vi "LDA_Beam_Alignment.vi"() -> ()   [LabVIEW 2014]
uses:
  Anemometry Sub Vis/Controls/Beam_Type.ctl
  Anemometry Sub Vis/Gen Trav/Traverse_cluster.ctl
  Anemometry Sub Vis/Gen Trav/Spacing.ctl
  Anemometry Sub Vis/Controls/Multi_run_mode.ctl
  Anemometry Sub Vis/Controls/User_Specific_mode.ctl
  Anemometry Sub Vis/Controls/Tunnel_Coordinates.ctl
  Anemometry Sub Vis/Controls/Post_Process.ctl
  Anemometry Sub Vis/Controls/Setup.ctl
  Anemometry Sub Vis/Gen Trav/Trav_mode.ctl
  Anemometry Sub Vis/Globals/Trav_pos_global.vi
  Anemometry Sub Vis/Globals/Meas_global.vi
  Anemometry Sub Vis/Globals/Preference_global.vi
panel:
  in  "Beams to peak":bool[](array[boolean])=[TRUE, TRUE, TRUE, TRUE]
  out "Beam Names":string[](array[string])
  out "Probe is facing...":string
  out "In-Plane Roll (deg)":dbl
  out "Pitch (deg)":dbl
  out "Yaw (deg)":dbl
  out "Vp (Actual Probe dir. vect)":dbl[](array[numeric])
  in  "Mode":T1(ring)
  out "Values Out":dbl[][](array[numeric])
  out "Original Position":dbl[](array[numeric]) format="%.2f"
  in  "Traverse Position":dbl[](array[numeric])=[0.0, 0.0, 0.0] format="%.2f"
  out "Message":string
  in  "Go Back":bool
  in  "OK":bool
  in  "stop":bool
  in  "Working On":T2 items=["Green Unshifted", "Green Shifted", "Blue Unshifted", "Blue Shifted"]
  # "X                 Y              Z"
  # "X                 Y              Z"
  # "Green Unshifted\nGreen Shifted\nBlue Unshifted\nBlue Shifted"
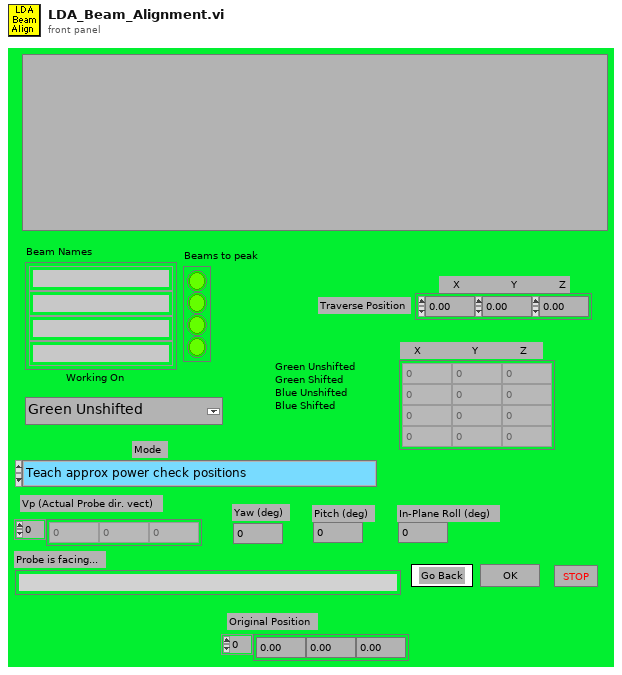
[diagram p1: front panel]
types:
  T1 = enum16{"Teach approx power check positions", "Hunt for optimum power check positions", "Check Beam powers now", "Peak up beam power using manipulators"}
  T2 = typedef "Beam_Type.ctl" = u16
  T3 = typedef "Traverse_cluster.ctl" = cluster{"Start X":dbl, "Start Y":dbl, "Start Z":dbl, "End X":dbl, "End Y":dbl, "End Z":dbl, "No. of pts.":i32, "Spacing":T4, "Filename":path, "Tunnel Speed":dbl, "Averaging time (min)":dbl, "Extra Commands":string, "Specific Arguments":string, "Emission Rate (l/min)":dbl, "Trace Gas Concentration (%)":dbl, "Density Ratio":string, "Comments":string, "Row No":i32, "Row Type Selector":T5, "Completion time":string, "Row Duration (mins)":dbl, "No. of Valid pts.":i32, "Meas Setup File":string}
  T4 = typedef "Spacing.ctl" = enum16{"Linear", "Log", "Gauss", "Specified", "N/A"}
  T5 = typedef "Multi_run_mode.ctl" = enum16{"Move Traverse Only", "Set Tunnel Speed Only", "Set Source Only", "Set Measurement Conditions", "Single Measurement", "Vertical Profile", "Lateral Profile", "Longitudinal Profile", "Explore Volume", "Multi-Axis Profile", "Auto Calibrate", "Meas Fast FID Bkgnd", "Check Beam Power", "Scanning Valve Measurement", "Run VI Named:", "Set ADAM Ch", "Wait (minutes)", "Send Message", "Synchronize With:", "Fall Back to this Row", "Turn Off Row Repeating", "Blank Row", "Traverse 3D Volume"}
  T6 = typedef "Tunnel_Coordinates.ctl" = enum16{"Work in Tunnel Coordinates", "Work in Model Coordinates"}
  T7 = typedef "User_Specific_mode.ctl" = enum16{"Check VI only", "Run VI"}
  T8 = typedef "Post_Process.ctl" = enum16{"Take New Data", "Post Process Raw Data File"}
  T9 = enum16{"Load setup from excel file", "Save setup to excel file"}
  T10 = enum16{"Load From Excel File", "Save to Excel File"}
  T11 = typedef "Setup.ctl" = enum16{"Run Program", "Show Setup", "Save Current Setup", "Setup Front Panel"}
  T12 = typedef "Trav_mode.ctl" = enum16{"Move traverse", "Read traverse position", "Teach Position"}
  T13 = typedef "LDA_Beam_Cluster.ctl" = cluster{"Vg1 (Green 1 dir. vect.)":dbl[], "Vg2  (Green 2 dir. vect.)":dbl[], "Vb1 (Blue 1 dir. vect.)":dbl[], "Vb2 (Blue 1 dir. vect.)":dbl[], "Porb (Orb XYZ posn. forced coplanar)":dbl[], "Porb (Orb XYZ posn. - allow skew)":dbl[], "Orb posn. uncertainty, +/- dx, dy, dz":dbl[], "Vp (Actual Probe dir. vect)":dbl[], "Yaw (deg)":dbl, "Pitch (deg)":dbl, "In-Plane Roll (deg)":dbl, "Beam Half Angle (deg)":dbl, "B1 Close P11":dbl[], "B1 Far P12":dbl[], "B2 Close P22":dbl[], "B2 Far P21":dbl[], "Projected Roll (deg)":dbl, "Green Velocity Vector":dbl[], "Blue Velocity Vector":dbl[], "Probe is facing....":string, "Calculation Method":string}
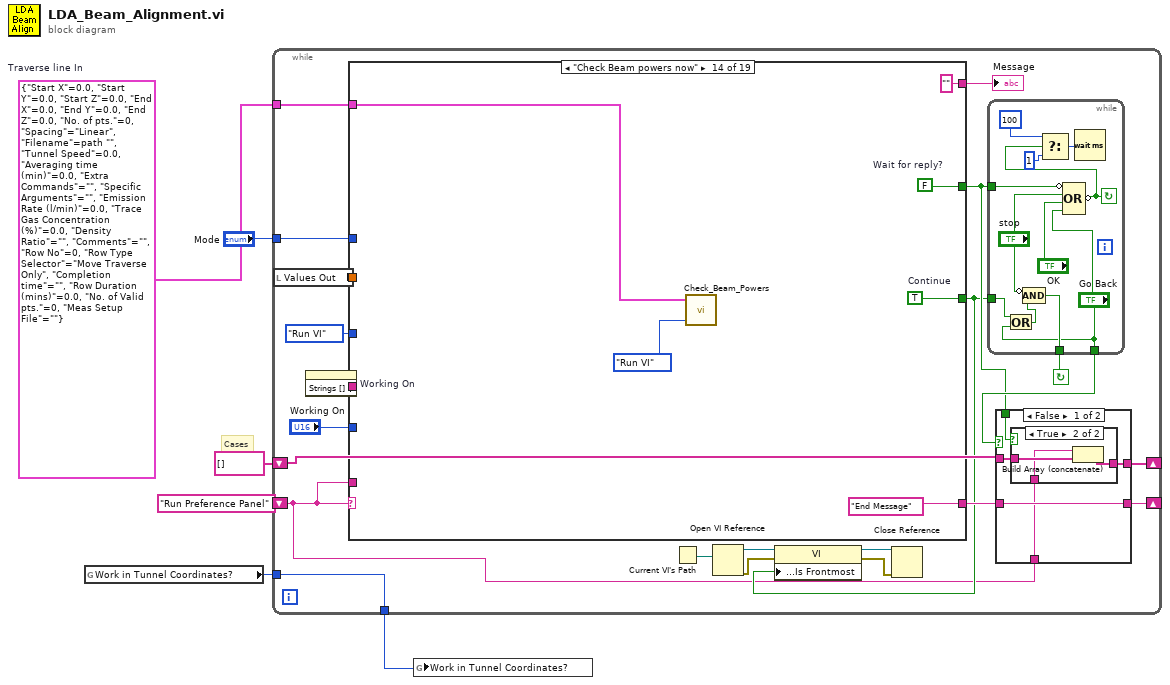
[diagram p0: block diagram]
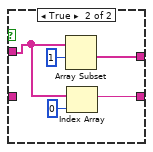
[diagram p3: hidden frame]
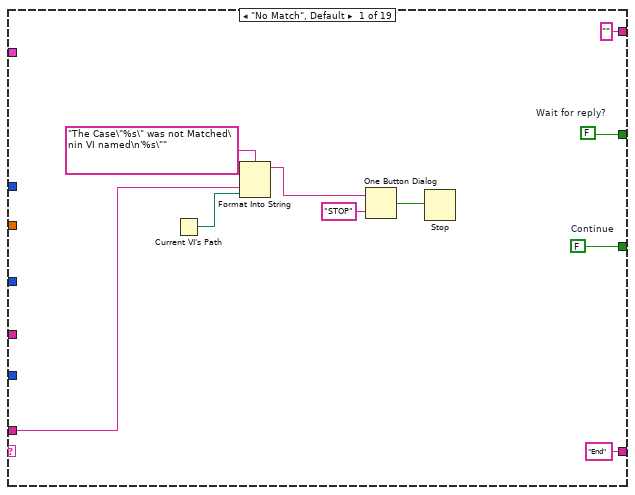
[diagram p4: hidden frame]
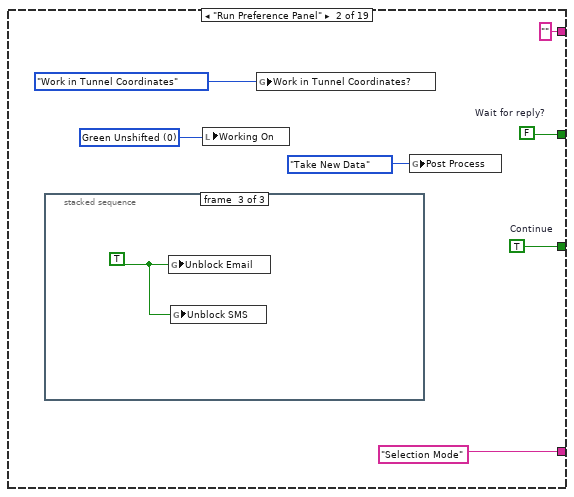
[diagram p5: hidden frame]
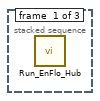
[diagram p6: hidden frame]
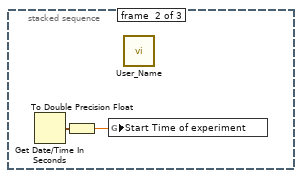
[diagram p7: hidden frame]
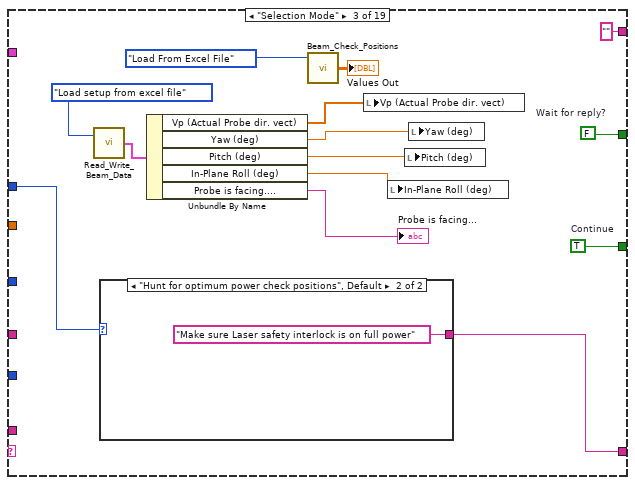
[diagram p8: hidden frame]
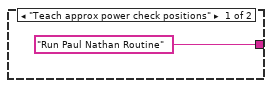
[diagram p9: hidden frame]
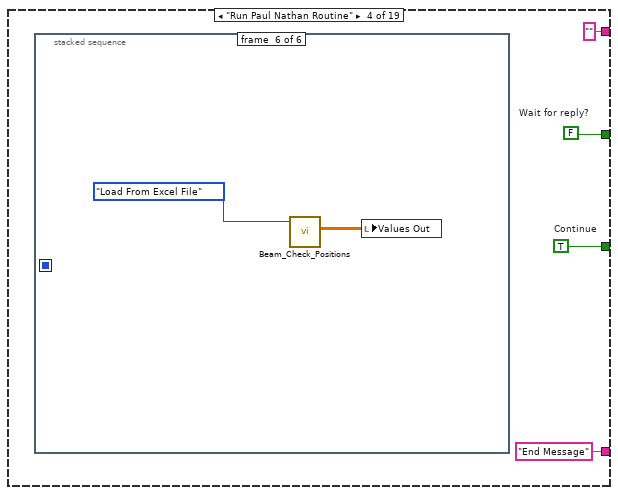
[diagram p10: hidden frame]
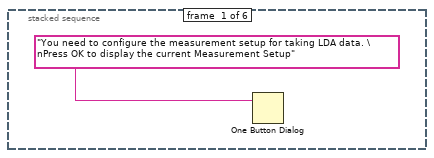
[diagram p11: hidden frame]
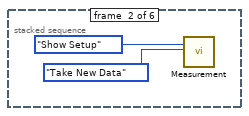
[diagram p12: hidden frame]
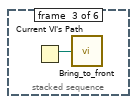
[diagram p13: hidden frame]
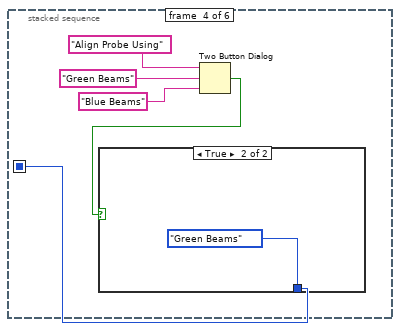
[diagram p14: hidden frame]
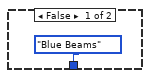
[diagram p15: hidden frame]
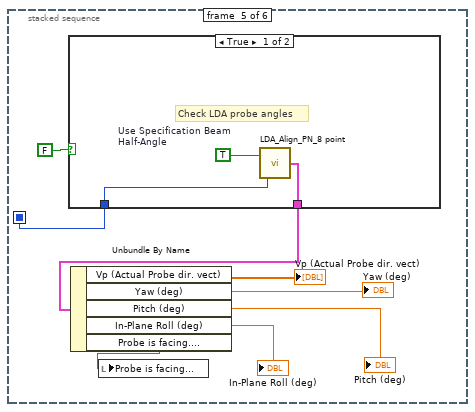
[diagram p16: hidden frame]
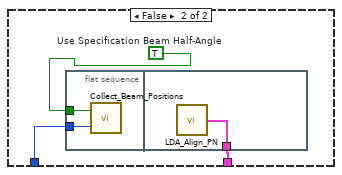
[diagram p17: hidden frame]
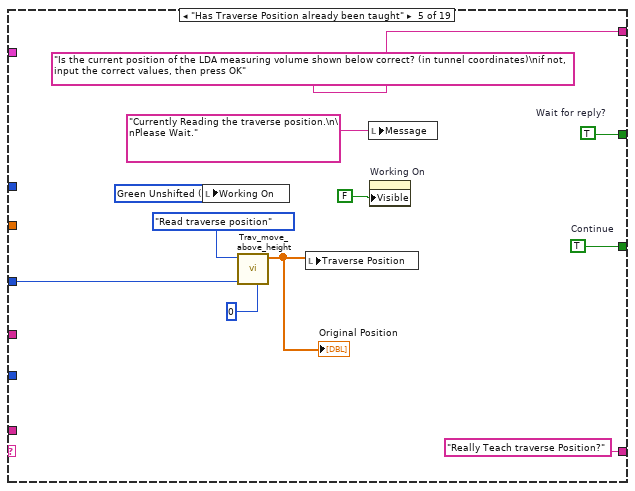
[diagram p18: hidden frame]
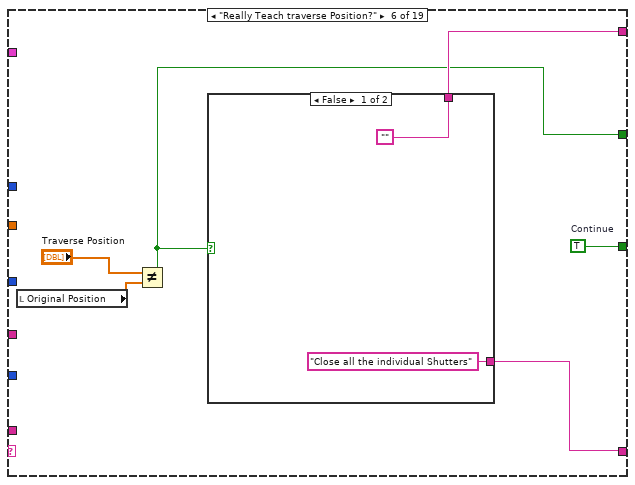
[diagram p19: hidden frame]
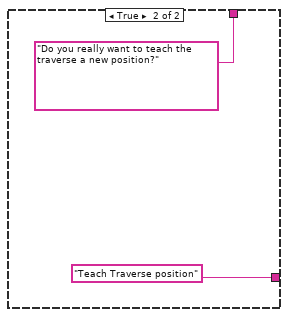
[diagram p20: hidden frame]
diagram:
  w3 = T3 {"Start X"=0.0, "Start Y"=0.0, "Start Z"=0.0, "End X"=0.0, "End Y"=0.0, "End Z"=0.0, "No. of pts."=0, "Spacing"=enum."Linear", "Filename"=path "", "Tunnel Speed"=0.0, "Averaging time (min)"=0.0, "Extra Commands"="", "Specific Arguments"="", "Emission Rate (l/min)"=0.0, "Trace Gas Concentration (%)"=0.0, "Density Ratio"="", "Comments"="", "Row No"=0, "Row Type Selector"=enum."Move Traverse Only", "Completion time"="", "Row Duration (mins)"=0.0, "No. of Valid pts."=0, "Meas Setup File"=""}  # Traverse line In
  # "Cases"
  n1 = global read "Trav_pos_global.vi" "Work in Tunnel Coordinates?"() -> (w1:T6)
  n2 = while {
    tunnel: w3 -> [w9]
    tunnel: "Mode" -> [w10]
    shift-left: string[] [] -> [w26]
    shift-right: [w25] -> _
    shift-left: "Run Preference Panel" -> [w8]
    shift-right: [w24] -> _
    tunnel: [w7] -> w2
    tunnel: w1 -> [w7]
    stop <- w28 continue-if-true
    n3 = local read "Values Out"() -> (w11:dbl[][])
    n4 = property on="Working On" class="Ring (strict)"() -> ("Strings []"=w13:string[])  [unwired: 2 in, 2 out]
    n5 = case shown="\"Check Beam powers now\"" w8 {
      tunnel: [w63 w70 w87 w93 w134 w140 w153 w163 w172 w188 w213 w223 w237 w263 w283 w287 w302 w310 w320] -> w14
      tunnel: ["End" "Selection Mode" w83 "End Message" "Really Teach traverse Position?" w135 "Close all the individual Shutters" "Manually move the traverse using hand wheels" "Read traverse position" w176 w207 "Hunt for optimum power check positions" "End Message" "End Message" "Read Beam Power" "Save measured beam Power" w294 "End Message" "End"] -> w23
      tunnel: [w62 w69 w86 w92 w133 w136 w152 w162 w171 w187 w212 w222 w238 w264 w282 w286 w301 w309 w319] -> w15
      tunnel: ["" "" "" "" "Is the current position of the LDA measuring volume shown below correct? (in tunnel coordinates)\nif not, input the correct values, then press OK" w139 "\"Teach Position\"\nHas been Executed" w156 w165 w173 "Make sure the Laser safety interlock is on full power and all the shutters are open." "Please select which beams you would like to hunt for optimum power check positions for by pressing the green buttons." "" "" w269 w285 w293 "Now open all the individual shutters so all four beam are showing." w313] -> w22
      tunnel: User_Specific_mode."Run VI" ("Simulate/Run") -> [_ _ _ _ w129 _ w148 _ _ w184 _ _ _ _ w279 _ _ _ _]
      tunnel: w13 -> [_ _ _ _ _ _ _ w161 w168 _ w210 w218 w226 _ w274 _ w290 _ _]
      tunnel: "Working On" -> [_ _ _ _ _ _ _ w160 w167 w175 w209 _ _ _ w273 _ w291 _ _]
      tunnel: w11 -> [_ _ _ _ _ _ _ _ _ w174 _ _ _ _ w272 _ w299 _ _]
      tunnel: w10 -> [_ _ w84 _ _ _ _ _ _ _ w208 _ _ _ _ _ _ _ w316]
      tunnel: w9 -> [_ _ _ _ _ _ _ _ _ _ _ _ _ w261 _ _ _ _ _]
      tunnel: w8 -> [w54 _ _ _ _ _ _ _ _ _ _ _ _ _ _ _ _ _ _]
      frame "No Match", Default {
        w62 = FALSE  # Wait for reply?
        w63 = FALSE  # Continue
        n6 = Current VI's Path() -> (path=w55:path)
        n7 = Format Into String(format string="The Case\"%s\" was not Matched\nin VI named\n'%s\"" ("Format String"), w54, w55) -> (resulting string=w58:string)  [unwired: 2 in, 1 out]
        n8 = One Button Dialog(message=w58, button name ("OK")="STOP") -> (true=w56:bool)
        n9 = Stop(stop? (T)=w56) -> ()
      }
      frame "Run Preference Panel" {
        w67 = T2 0 items=["Green Unshifted", "Green Shifted", "Blue Unshifted", "Blue Shifted"] ("Beam Type")
        w69 = FALSE  # Wait for reply?
        w70 = TRUE  # Continue
        n10 = stacked-sequence {
          frame #0 {
            n11 = call "Run_EnFlo_Hub.vi"() -> ()  [unwired: 8 out]
          }
          frame #1 {
            n12 = Get Date/Time In Seconds() -> (seconds since 1Jan1904=w72:timestamp)
            n13 = To Double Precision Float(number=w72) -> (double precision float=w71:dbl)
            n14 = global write "Meas_global.vi" "Start Time of experiment"(w71) -> ()
            n15 = call "User_Name.vi"() -> ()  [unwired: 1 out]
          }
          frame #2 {
            w73 = TRUE
            n16 = global write "Preference_global.vi" "Unblock Email"(w73) -> ()
            n17 = global write "Preference_global.vi" "Unblock SMS"(w73) -> ()
          }
        }
        n18 = local write "Working On"(w67) -> ()
        n19 = global write "Trav_pos_global.vi" "Work in Tunnel Coordinates?"(Tunnel_Coordinates."Work in Tunnel Coordinates" ("Work in Tunnel Coordinates?")) -> ()
        n20 = global write "Meas_global.vi" "Post Process"(Post_Process."Take New Data" ("Post Process")) -> ()
      }
      frame "Selection Mode" {
        w86 = FALSE  # Wait for reply?
        w87 = TRUE  # Continue
        n21 = call "Read_Write_Beam_Data.vi"("Mode"=T9."Load setup from excel file") -> ("Beam Data Out"=w75:T13)  [unwired: 1 in]
        n22 = case shown="\"Hunt for optimum power check positions\", Default" w84 {
          tunnel: ["Run Paul Nathan Routine" "Make sure Laser safety interlock is on full power"] -> w83
          frame "Teach approx power check positions" {
          }
          frame "Hunt for optimum power check positions", Default {
          }
        }
        n23 = Unbundle By Name(w75) -> ("Vp (Actual Probe dir. vect)"=w80:dbl[], "Yaw (deg)"=w77:dbl, "Pitch (deg)"=w78:dbl, "In-Plane Roll (deg)"=w79:dbl, "Probe is facing...."=→"Probe is facing...":string)
        n24 = call "Beam_Check_Positions.vi"("Mode"=T10."Load From Excel File") -> ("Values Out"=→"Values Out":dbl[][])  [unwired: 1 in, 1 out]
        n25 = local write "Vp (Actual Probe dir. vect)"(w80) -> ()
        n26 = local write "In-Plane Roll (deg)"(w79) -> ()
        n27 = local write "Pitch (deg)"(w78) -> ()
        n28 = local write "Yaw (deg)"(w77) -> ()
      }
      frame "Run Paul Nathan Routine" {
        w92 = FALSE  # Wait for reply?
        w93 = TRUE  # Continue
        n29 = stacked-sequence {
          seq-local: [_ _ _ w98 _ _] -> [_ _ _ _ w106 _]
          frame #0 {
            n30 = One Button Dialog(message="You need to configure the measurement setup for taking LDA data. \nPress OK to display the current Measurement Setup") -> ()  [unwired: 1 in, 1 out]
          }
          frame #1 {
            n31 = call "Measurement.vi"("setup"=Setup."Show Setup", "Post Process"=Post_Process."Take New Data") -> ()  [unwired: 16 in, 2 out]
          }
          frame #2 {
            n32 = Current VI's Path() -> (path=w97:path)
            n33 = call "Bring_to_front.vi"("path"=w97) -> ()
          }
          frame #3 {
            n34 = Two Button Dialog(message="Align Probe Using", 1:"Blue Beams" ("F button name (\"Cancel\")"), 2:"Green Beams" ("T button name (\"OK\")")) -> (T button?=w99:bool)
            n35 = case shown="True" w99 {
              tunnel: [enum16{"Green Beams", "Blue Beams"}."Blue Beams" ("Align Probe Using") enum16{"Green Beams", "Blue Beams"}."Green Beams" ("Align Probe Using")] -> w98
              frame False {
              }
              frame True {
              }
            }
          }
          frame #4 {
            n36 = case shown="True" FALSE ("Case Constant\n(See Context Help)") {
              tunnel: [w114 w116] -> w112
              tunnel: w106 -> [w113 w118]
              frame True {
                w115 = TRUE  # Use Specification Beam Half-Angle
                # "Check LDA probe angles"
                n37 = call "LDA_Align_PN_8 point.vi"("Align Probe Using"=w113, "Use Specification Beam Half-Angle"=w115) -> ("Beam Data"=w114:T13)
              }
              frame False {
                w117 = TRUE  # Use Specification Beam Half-Angle
                n38 = flat-sequence {
                  tunnel: w118 -> [w120]
                  tunnel: w117 -> [w119]
                  tunnel: [w121] -> w116
                  frame #0 {
                    n39 = call "Collect_Beam_Positions.vi"("Align Probe Using"=w120, "Use Specification Beam Half-Angle"=w119) -> ()  [unwired: 1 out]
                  }
                  frame #1 {
                    n40 = call "LDA_Align_PN.vi"() -> ("Beam Data"=w121:T13)  [unwired: 2 in]
                  }
                }
              }
            }
            n41 = Unbundle By Name(w112) -> ("Vp (Actual Probe dir. vect)"=→"Vp (Actual Probe dir. vect)":dbl[], "Yaw (deg)"=→"Yaw (deg)":dbl, "Pitch (deg)"=→"Pitch (deg)":dbl, "In-Plane Roll (deg)"=→"In-Plane Roll (deg)":dbl, "Probe is facing...."=w107:string)
            n42 = local write "Probe is facing..."(w107) -> ()
          }
          frame #5 {
            n43 = call "Beam_Check_Positions.vi"("Mode"=T10."Load From Excel File") -> ("Values Out"=w122:dbl[][])  [unwired: 1 in, 1 out]
            n44 = local write "Values Out"(w122) -> ()
          }
        }
      }
      frame "Has Traverse Position already been taught" {
        w127 = T2 0 items=["Green Unshifted", "Green Shifted", "Blue Unshifted", "Blue Shifted"] ("Beam Type")
        w133 = TRUE  # Wait for reply?
        w134 = TRUE  # Continue
        n45 = local write "Working On"(w127) -> ()
        n46 = call "Trav_move_above_height.vi"("Currently on Point"=0, "Simulate/Run"=w129, "Mode"=Trav_mode."Read traverse position") -> ("Trav Position achieved"=w128:dbl[])  [unwired: 5 in, 3 out]
        "Original Position" <- w128
        n47 = local write "Traverse Position"(w128) -> ()
        n48 = local write "Message"("Currently Reading the traverse position.\n\nPlease Wait." ("Message")) -> ()
        n49 = property on="Working On" class="Ring (strict)"("Visible"=FALSE ("Write Attribute")) -> ()  [unwired: 2 in, 2 out]
      }
      frame "Really Teach traverse Position?" {
        w140 = TRUE  # Continue
        n50 = local read "Original Position"() -> (w138:dbl[])
        n51 = Not Equal?(x="Traverse Position", y=w138) -> (x != y?=w136:bool)
        n52 = case shown="False" w136 {
          tunnel: ["" "Do you really want to teach the traverse a new position?"] -> w139
          tunnel: ["Close all the individual Shutters" "Teach Traverse position"] -> w135
          frame False {
          }
          frame True {
          }
        }
      }
      frame "Teach Traverse position" {
        w152 = FALSE  # Wait for reply?
        w153 = TRUE  # Continue
        n53 = local read "Traverse Position"() -> (w147:dbl[])
        n54 = call "Trav_move_above_height.vi"("Currently on Point"=0, "Simulate/Run"=w148, "New Position"=w147, "Mode"=Trav_mode."Teach Position") -> ()  [unwired: 4 in, 4 out]
        n55 = local write "Message"("Currently Teaching the traverse position.\n\nPlease Wait" ("Message")) -> ()
      }
      frame "Close all the individual Shutters" {
        w162 = TRUE  # Wait for reply?
        w163 = TRUE  # Continue
        n56 = Index Array(array=w161, index=w160) -> (element=w159:string)
        n57 = Format Into String(format string="Close all the individual shutters except for the %s laser beam.", w159) -> (resulting string=w156:string)  [unwired: 2 in, 1 out]
        n58 = property on="Working On" class="Ring (strict)"("Visible"=TRUE ("Write Attribute"), "Disabled"=u8 0 ("Write Attribute")) -> ()  [unwired: 2 in, 2 out]
      }
      frame "Manually move the traverse using hand wheels" {
        w171 = TRUE  # Wait for reply?
        w172 = TRUE  # Continue
        n59 = Index Array(array=w168, index=w167) -> (element=w169:string)
        n60 = property on="Working On" class="Ring (strict)"("Disabled"=u8 1 ("Write Attribute")) -> ()  [unwired: 2 in, 2 out]
        n61 = Format Into String(format string="Go into the tunnel and manually move the traverse using the hand wheels so that the %s laser beam is pointing at the center of the light sensor.\n", w169) -> (resulting string=w165:string)  [unwired: 2 in, 1 out]
      }
      frame "Read traverse position" {
        w178 = T2 3 items=["Green Unshifted", "Green Shifted", "Blue Unshifted", "Blue Shifted"] ("Beam Type")
        w173 = "Currently Reading the traverse Position.\n\nPlease Wait"
        w187 = FALSE  # Wait for reply?
        w188 = TRUE  # Continue
        n62 = To Long Integer(number=w175) -> (32bit integer=w183:i32)
        n63 = call "Trav_move_above_height.vi"("Currently on Point"=0, "Simulate/Run"=w184, "Mode"=Trav_mode."Read traverse position") -> ("Trav Position achieved"=w182:dbl[])  [unwired: 5 in, 3 out]
        n64 = for {
          N: 4 -> [_]
          tunnel: w174 -> [w199]
          tunnel: w183 -> [w197]
          tunnel: [w195] -> w179 mode=indexing
          tunnel: w182 -> [w193]
          i -> [w198]
          n65 = Index Array(array=w199, index (row)=w198) -> (element=w194:dbl[])  [unwired: 1 in]
          n66 = Equal?(x=w198, y=w197) -> (x = y?=w196:bool)
          n67 = case shown="True" w196 {
            tunnel: [w200 w203] -> w195
            tunnel: w194 -> [w200 w205]
            tunnel: w193 -> [_ w201]
            frame False {
            }
            frame True {
              n68 = Index Array(array=w205, index=3 ("Index")) -> (element=w202:dbl)
              n69 = Build Array (concatenate)(w201, w202) -> (w203:dbl[])
            }
          }
        }
        n70 = Equal?(x=w175, y=w178) -> (x = y?=w177:bool)
        n71 = case shown="False" w177 {
          tunnel: ["Close all the individual Shutters" "Open all individual laser shutters again"] -> w176
          tunnel: w175 -> [w190 _]
          frame False {
            n72 = Increment(x=w190) -> (x+1=w191:T2)
            n73 = local write "Working On"(w191) -> ()
          }
          frame True {
          }
        }
        n74 = local write "Values Out"(w179) -> ()
        n75 = local write "Message"(w173) -> ()
        n76 = call "Beam_Check_Positions.vi"("Values"=w179, "Mode"=T10."Save to Excel File") -> ()  [unwired: 2 out]
      }
      frame "Make sure Laser safety interlock is on full power" {
        w212 = TRUE  # Wait for reply?
        w213 = TRUE  # Continue
        n77 = Index Array(array=w210, index=w209) -> ()  [unwired: 1 out]
        n78 = property on="Working On" class="Ring (strict)"("Disabled"=u8 1 ("Write Attribute")) -> ()  [unwired: 2 in, 2 out]
        n79 = case shown="\"Hunt for optimum power check positions\"" w208 {
          tunnel: ["Has Traverse Position already been taught" "Find Peak for which beams?" "Check Beam powers now" "Move Traverse to next Meas position"] -> w207
          frame "Teach approx power check positions" {
          }
          frame "Hunt for optimum power check positions" {
          }
          frame "Check Beam powers now" {
          }
          frame "Peak up beam power using manipulators" {
          }
        }
      }
      frame "Find Peak for which beams?" {
        w222 = TRUE  # Wait for reply?
        w223 = TRUE  # Continue
        n80 = property on="Working On" class="Ring (strict)"("Disabled"=u8 1 ("Write Attribute")) -> ()  [unwired: 2 in, 2 out]
        "Beam Names" <- w218
      }
      frame "Hunt for optimum power check positions" {
        w238 = FALSE  # Wait for reply?
        w237 = TRUE  # Continue
        w243 = T3 {"Start X"=0.0, "Start Y"=0.0, "Start Z"=0.0, "End X"=0.0, "End Y"=0.0, "End Z"=0.0, "No. of pts."=0, "Spacing"=enum."Linear", "Filename"=path "", "Tunnel Speed"=0.0, "Averaging time (min)"=0.0, "Extra Commands"="", "Specific Arguments"="", "Emission Rate (l/min)"=0.0, "Trace Gas Concentration (%)"=0.0, "Density Ratio"="", "Comments"="", "Row No"=0, "Row Type Selector"=enum."Move Traverse Only", "Completion time"="", "Row Duration (mins)"=0.0, "No. of Valid pts."=0, "Meas Setup File"=""}  # Traverse line In
        w229 = 0.85 ("y")
        n81 = local read "Vp (Actual Probe dir. vect)"() -> (w235:dbl[])
        n82 = for {
          shift-right: [w247] -> w225
          shift-left: "; " -> [w246]
          tunnel: "Beams to peak" -> [w248] mode=indexing
          tunnel: w226 -> [w245] mode=indexing
          n83 = case shown="True" w248 {
            tunnel: [w249 w253] -> w247
            tunnel: w246 -> [w249 w252]
            tunnel: w245 -> [_ w251]
            frame False {
            }
            frame True {
              n84 = Concatenate Strings(w252, w251, ";  " ("string")) -> (w253:string)
            }
          }
        }
        n85 = Absolute Value(x=w235) -> (abs(x)=w234:dbl[])
        n86 = Array To Cluster(array=w234) -> (cluster=w233:cluster{"[0]":dbl, "[1]":dbl, "[2]":dbl})
        n87 = Unbundle(w233) -> ("[0]"=w232:dbl, "[1]"=w230:dbl)  [unwired: 1 out]
        n88 = Greater?(x=w232, y=w229) -> (0:w231:bool)
        n89 = case shown="True" w231 {
          tunnel: [w257 "X Axis Fixed"] -> w244
          tunnel: w230 -> [w256 _]
          tunnel: w229 -> [w255 _]
          frame False {
            n90 = Greater?(x=w256, y=w255) -> (0:w254:bool)
            n91 = case shown="False" w254 {
              tunnel: ["Z Axis Fixed" "Y Axis Fixed"] -> w257
              frame False {
              }
              frame True {
              }
            }
          }
          frame True {
          }
        }
        n92 = Concatenate Strings("First Argument;" ("string"), w244, w225) -> (w242:string)
        n93 = Bundle By Name(cluster=w243, "Specific Arguments"=w242) -> (w241:T3)
        n94 = call "Find_Beam_Max_Pos.vi"("Mode"=User_Specific_mode."Run VI", "Traverse line In"=w241) -> ()  [unwired: 4 out]
      }
      frame "Check Beam powers now" {
        w264 = FALSE  # Wait for reply?
        w263 = TRUE  # Continue
        n95 = call "Check_Beam_Powers.vi"("Mode"=User_Specific_mode."Run VI", "Traverse line In"=w261) -> ()  [unwired: 1 in, 3 out]
      }
      frame "Move Traverse to next Meas position" {
        w282 = FALSE  # Wait for reply?
        w283 = TRUE  # Continue
        n96 = Index Array(array=w274, index=w273) -> (element=w267:string)
        n97 = Format Into String(format string="The %s laser beam should now be hitting the light sensor. Please Peak up this beam to achieve the maximum output", w267) -> (resulting string=w269:string)  [unwired: 2 in, 1 out]
        n98 = Format Into String(format string="Currently moving Traverse.\n\nThe %s Laser Beam should soon be hitting the light sensor.\n\nPlease Wait", w267) -> (resulting string=w271:string)  [unwired: 2 in, 1 out]
        n99 = call "PM100D_Plot_ph.vi"("Beam Name"=w267) -> ()  [unwired: 1 out]
        n100 = Index Array(array=w272, index (row)=w273) -> (element=w278:dbl[])  [unwired: 1 in]
        n101 = local write "Message"(w271) -> ()
        n102 = Array Subset(array=w278, length=3 ("Array Length")) -> (w276:dbl[])  [unwired: 1 in]
        n103 = call "Trav_move_above_height.vi"("Currently on Point"=0, "Simulate/Run"=w279, "New Position"=w276, "Mode"=Trav_mode."Move traverse") -> ()  [unwired: 4 in, 4 out]
      }
      frame "Read Beam Power" {
        w285 = "Currently Reading the Beam Power\n\nPlease Wait"
        w286 = FALSE  # Wait for reply?
        w287 = TRUE  # Continue
        n104 = local write "Message"(w285) -> ()
      }
      frame "Save measured beam Power" {
        w296 = T2 3 items=["Green Unshifted", "Green Shifted", "Blue Unshifted", "Blue Shifted"] ("Beam Type")
        w293 = "Writing Beam Power to file"
        w301 = FALSE  # Wait for reply?
        w302 = TRUE  # Continue
        n105 = Index Array(array=w290, index=w291) -> (element=w289:string)
        n106 = Equal?(x=w291, y=w296) -> (x = y?=w295:bool)
        n107 = call "PM100D_Single_Value_ph.vi"("Averaging Period (s)"=3.0, "Beam Name"=w289) -> ("Light Power mW"=w292:dbl)  [unwired: 1 out]
        n108 = case shown="False" w295 {
          tunnel: ["Move Traverse to next Meas position" "End Message"] -> w294
          tunnel: w291 -> [w305 _]
          frame False {
            n109 = Increment(x=w305) -> (x+1=w304:T2)
            n110 = local write "Working On"(w304) -> ()
          }
          frame True {
          }
        }
        n111 = Replace Array Subset(array=w299, new element=w292, index (row)=w291, index (col)=3 ("Index")) -> (w297:dbl[][])
        n112 = local write "Message"(w293) -> ()
        n113 = local write "Values Out"(w297) -> ()
        n114 = call "Beam_Check_Positions.vi"("Values"=w297, "Mode"=T10."Save to Excel File") -> ()  [unwired: 2 out]
      }
      frame "Open all individual laser shutters again" {
        w309 = TRUE  # Wait for reply?
        w310 = TRUE  # Continue
      }
      frame "End Message" {
        w319 = FALSE  # Wait for reply?
        w320 = FALSE  # Continue
        n115 = property on="Mode" class="Enum (strict)"() -> ("Strings []"=w317:string[])  [unwired: 2 in, 2 out]
        n116 = Index Array(array=w317, index=w316) -> (element=w315:string)
        n117 = Format Into String(format string="%s\nhas now been completed" ("Format String"), w315) -> (resulting string=w313:string)  [unwired: 2 in, 1 out]
        n118 = call "Beam_Check_Positions.vi"("Mode"=T10."Load From Excel File") -> ("Values Out"=w311:dbl[][])  [unwired: 1 in, 1 out]
        n119 = local write "Values Out"(w311) -> ()
      }
    }
    "Message" <- w22
    n120 = Current VI's Path() -> (path=w20:path)
    n121 = Open VI Reference(vi path=w20) -> (vi reference=w19:refnum<vi>, error out=w18:errorcluster)  [unwired: 1 in, 4 out]
    n122 = property class="VI"(reference=w19, error in=w18, "Front Panel Window:Is Frontmost"=w14) -> (reference out=w17:refnum<vi>, error out=w16:errorcluster)
    n123 = Close Reference(reference=w17, error in (no error)=w16) -> ()  [unwired: 1 out]
    n124 = while {
      tunnel: ["Go Back"] -> w27
      tunnel: [w36] -> w28
      tunnel: w14 -> [w35]
      tunnel: w15 -> [w38]
      stop <- w32 continue-if-true
      n125 = Or(x=w35, y="Go Back") -> (x .or. y?=w33:bool)
      n126 = Compound Arithmetic op=AND(invert "stop", w33) -> (w36:bool)
      n127 = Compound Arithmetic op=OR(invert w38, "stop", "OK", "Go Back") -> (invert w32:bool)
      n128 = Select(t=u32 100 ("millisecond timer value"), s=w32, f=u32 1) -> (s? t:f=w29:u32)
      n129 = Wait (ms)(milliseconds to wait=w29) -> ()  [unwired: 1 out]
    }
    n130 = case shown="False" w27 {
      tunnel: w26 -> [w44 w49]
      tunnel: [w43 w50] -> w25
      tunnel: w8 -> [w41 _]
      tunnel: [w42 w51] -> w24
      tunnel: w23 -> [w42 _]
      tunnel: w15 -> [w40 _]
      frame False {
        n131 = case shown="True" w40 {
          tunnel: w44 -> [w45 w48]
          tunnel: [w45 w47] -> w43
          tunnel: w41 -> [_ w46]
          frame False {
          }
          frame True {
            n132 = Build Array (concatenate)(w46, w48) -> (w47:string[])
          }
        }
      }
      frame True {
        n133 = Array Subset(array=w49, index=1 ("Array Index")) -> (w50:string[])  [unwired: 1 in]
        n134 = Index Array(array=w49, index=0 ("Index")) -> (element=w51:string)
      }
    }
  }
  n135 = global write "Trav_pos_global.vi" "Work in Tunnel Coordinates?"(w2) -> ()
